vi "Global Stop.vi"() -> ()   [LabVIEW 2013]
panel:
  in  "Global Stop":bool
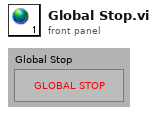
[diagram p1: front panel]
diagram:
